vi "Unpack (if allowable).vi"(11 "ObserverSet in":refnum<class "ObserverSet.lvclass">) -> (2 "Array out":refnum<class "Send.lvclass">[](array[class]))   [LabVIEW 2011, in "Messenging.lvlib" / "ObserverSet.lvclass"]
uses:
  ObserverSet.lvclass
  Send/Send.lvclass
  Message Translation/Translator/Translator.lvclass
  ObserverSet.lvclass/ObserverSet.ctl
  SendOnly/Observer.lvclass
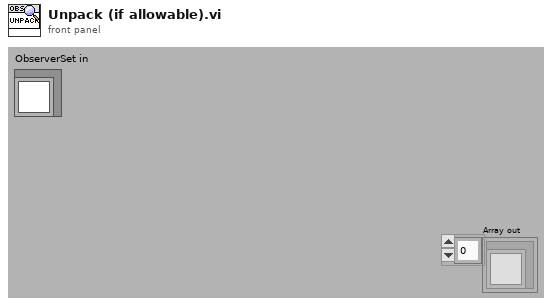
[diagram p1: front panel]
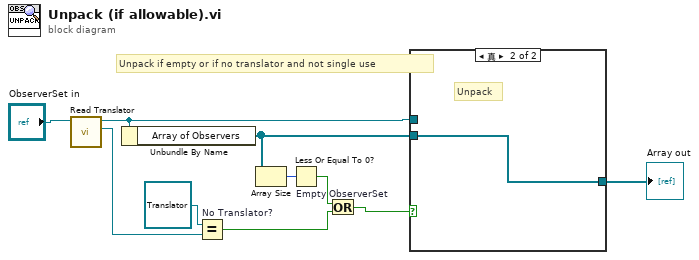
[diagram p0: block diagram]
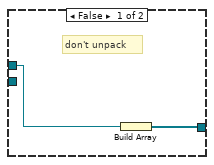
[diagram p2: hidden frame]
diagram:
  # "Unpack if empty or if no translator and not single use"
  n1 = call "Read Translator.vi"("Observer.lvclass in"="ObserverSet in") -> ("Messenging.lvlib:Translator.lvclass"=w9:refnum<class "Translator.lvclass">, "Observer.lvclass out"=w2:refnum<class "ObserverSet.lvclass">)  [unwired: 1 in, 8 out]
  n2 = Unbundle By Name(w2) -> ("Array of Observers"=w3:refnum<class "Send.lvclass">[])
  n3 = Equal? "No Translator?"(x=refnum<class "Translator.lvclass"> refnum ("Messenging.lvlib:Translator.lvclass"), y=w9) -> (x = y?=w1:bool)
  n4 = Array Size(array=w3) -> (size(s)=w7:i32)
  n5 = Less Or Equal To 0? "Empty ObserverSet"(x=w7) -> (x <= 0?=w5:bool)
  n6 = Or(x=w5, y=w1) -> (x .or. y?=w6:bool)
  n7 = case shown="真" w6 {
    tunnel: [w11 w13] -> w4
    tunnel: w3 -> [_ w13]
    tunnel: w2 -> [w12 _]
    frame False {
      # "don't unpack"
      n8 = Build Array(w12) -> (w11:refnum<class "ObserverSet.lvclass">[])
    }
    frame True {
      # "Unpack"
    }
  }
  "Array out" <- w4
